vi "Get status.vi"(8 "error in (no error)":errorcluster, 11 "Motor in":refnum<class "Motor.lvclass">) -> (0 "error out":errorcluster, 2 "status string":string, 3 "Motor out":refnum<class "Motor.lvclass">)   [LabVIEW 2018, in "Motor.lvclass"]
doc: "TESTE DOCUMENTA敲O"
uses:
  Motor.lvclass
  Motor.lvclass/Motor.ctl
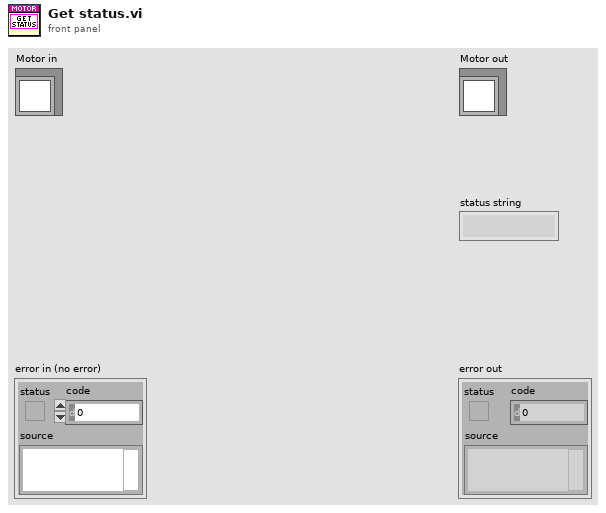
[diagram p1: front panel]
types:
  T1 = cluster{"action":string, "param":string, "pos_name":string, "pos_idx":i32, "ack":bool, "stop":bool, "offset":bool, "immediate":bool, "instructions":string[]}
  T2 = cluster{"mode":string, "condition":string, "position":string, "pos_name":string, "pos_id":string}
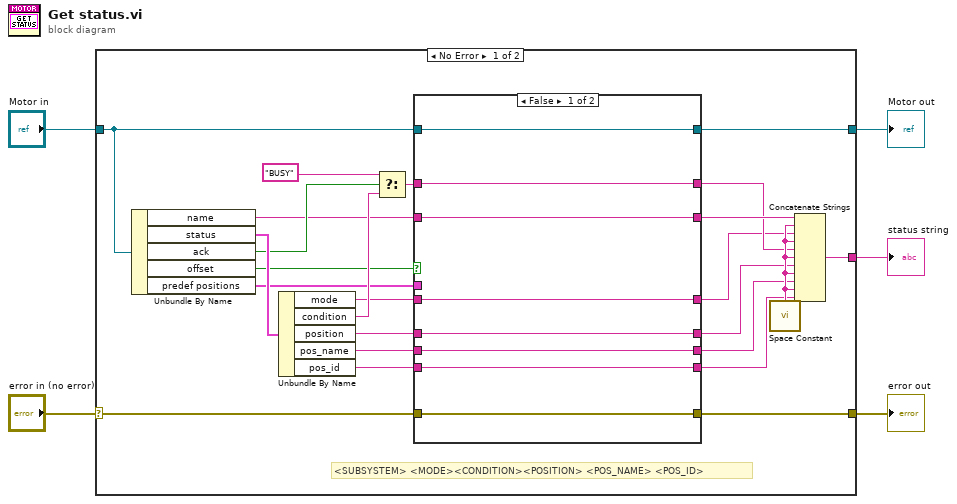
[diagram p0: block diagram]
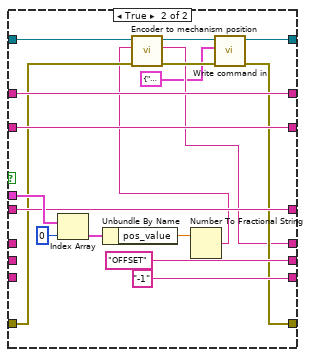
[diagram p2: hidden frame]
diagram:
  n1 = case shown="No Error" "error in (no error)" {
    selector: "error in (no error)" -> [w11 w56]
    tunnel: [w12 w56] -> w4
    tunnel: [w14 w57] -> w2
    tunnel: "Motor in" -> [w13 w57]
    tunnel: [w27 _] -> w1
    frame No Error {
      # "<SUBSYSTEM> <MODE><CONDITION><POSITION> <POS_NAME> <POS_ID>"
      n2 = Unbundle By Name(w13) -> ("name"=w8:string, "status"=w28:T2, "ack"=w17:bool, "offset"=w18:bool, "predef positions"=w16:cluster{"pos_name":string, "pos_value":dbl}[])
      n3 = Unbundle By Name(w28) -> ("mode"=w15:string, "condition"=w26:string, "position"=w21:string, "pos_name"=w20:string, "pos_id"=w19:string)
      n4 = Select(t="BUSY", s=w17, f=w26) -> (s? t:f=w10:string)
      n5 = case shown="False" w18 {
        tunnel: [w37 w39] -> w24
        tunnel: [w36 "OFFSET" ("t")] -> w23
        tunnel: [w35 "-1" ("t")] -> w22
        tunnel: w21 -> [w37 _]
        tunnel: w20 -> [w36 _]
        tunnel: w19 -> [w35 _]
        tunnel: w16 -> [_ w52]
        tunnel: w15 -> [w33 w48]
        tunnel: [w30 w51] -> w14
        tunnel: w13 -> [w30 w46]
        tunnel: [w34 w47] -> w12
        tunnel: w11 -> [w34 w45]
        tunnel: [w33 w48] -> w6
        tunnel: w10 -> [w31 w50]
        tunnel: [w32 w49] -> w9
        tunnel: w8 -> [w32 w49]
        tunnel: [w31 w50] -> w7
        frame False {
        }
        frame True {
          n6 = Index Array(array=w52, index=0) -> (element=w42:cluster{"pos_name":string, "pos_value":dbl})
          n7 = Unbundle By Name(w42) -> ("pos_value"=w41:dbl)
          n8 = Number To Fractional String(number=w41) -> (F-format string=w40:string)  [unwired: 3 in]
          n9 = call-dynamic "Encoder to mechanism position.vi"("error in (no error)"=w45, "motor position"=w40, "Motor in"=w46) -> ("error out"=w43:errorcluster, "mechanism position"=w39:string, "Motor out"=w44:refnum<class "Motor.lvclass">)  [unwired: 6 in]
          n10 = call-dynamic "Write command in.vi"("error in (no error)"=w43, "command in"=T1 {"action"="", "param"="", "pos_name"="", "pos_idx"=0, "ack"=FALSE, "stop"=FALSE, "offset"=FALSE, "immediate"=FALSE, "instructions"=[]}, "Motor in"=w44) -> ("error out"=w47:errorcluster, "Motor out"=w51:refnum<class "Motor.lvclass">)  [unwired: 7 in]
        }
      }
      n11 = call <vilib>:"Space Constant.vi"() -> ("String"=w29:string)
      n12 = Concatenate Strings(w9, w29, w6, w29, w7, w29, w24, w29, w23, w29, w22) -> (w27:string)
    }
    frame Error {
    }
  }
  "error out" <- w4
  "Motor out" <- w2
  "status string" <- w1
